vi "Memory.Pointer.Copy All.vi"   [LabVIEW 2016, in "Memory Manager.lvlib" / "Memory.Pointer.lvclass"]
uses:
  Memory.Pointer.lvclass
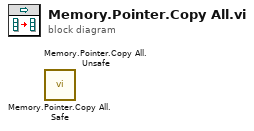
[diagram p0: block diagram]
diagram:
  n1 = call "Memory.Pointer.Copy All.Safe.vi"() -> ()  [unwired: 9 in, 3 out]
  n2 = call "Memory.Pointer.Copy All.Unsafe.vi"() -> ()  [unwired: 9 in, 3 out]
